vi "Puff_Analysis_AN.vi"(6 "Input Peak":dbl, 7 "Input Own Peak Value?":bool, 8 "Concentration":dbl[](array[numeric]), 9 "Time":dbl[](array[numeric])) -> (0 "End Index":i32, 1 "Start Index":i32, 2 "Channel Values":string[](array[string]), 3 "Channel Names":string[](array[string]))   [LabVIEW 2022 SP3]
uses:
  <vilib>/Analysis/6fits.llb/Curve Fitting Criteria.ctl
  <vilib>/Analysis/baseanly.llb/Mean (DBL).vi
  <vilib>/Analysis/NI_AALBase.lvlib
  <vilib>/Analysis/NI_AALPro.lvlib
panel:
  out "% Error":dbl
  out "offset":dbl
  out "Decay Constant (s)":dbl
  out "Start":dbl
  out "End":dbl
  out "XY Graph":cluster{"Time":dbl[], "Concentration":dbl[]}[](graph)
  out "Decay Time":dbl
  out "50-50 Time":dbl
  out "Rise Time":dbl
  out "Fall Times":dbl[](array[numeric])
  out "Rise Times":dbl[](array[numeric])
  out "Peak Value":dbl
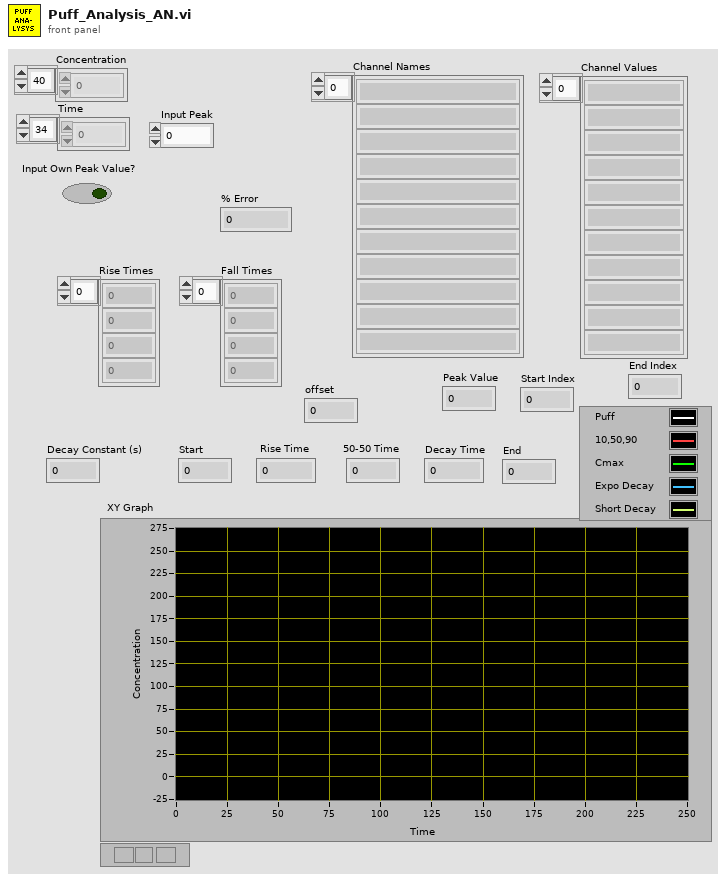
[diagram p1: front panel]
types:
  T1 = cluster{"amp min":dbl, "amp max":dbl, "damping min":dbl, "damping max":dbl, "offset min":dbl, "offset max":dbl}
  T2 = typedef "NI_AALPro.lvlib/Curve Fitting Criteria.ctl" = u16
  T3 = cluster{"Time":dbl[], "Best Exponential Fit":dbl[]}[]
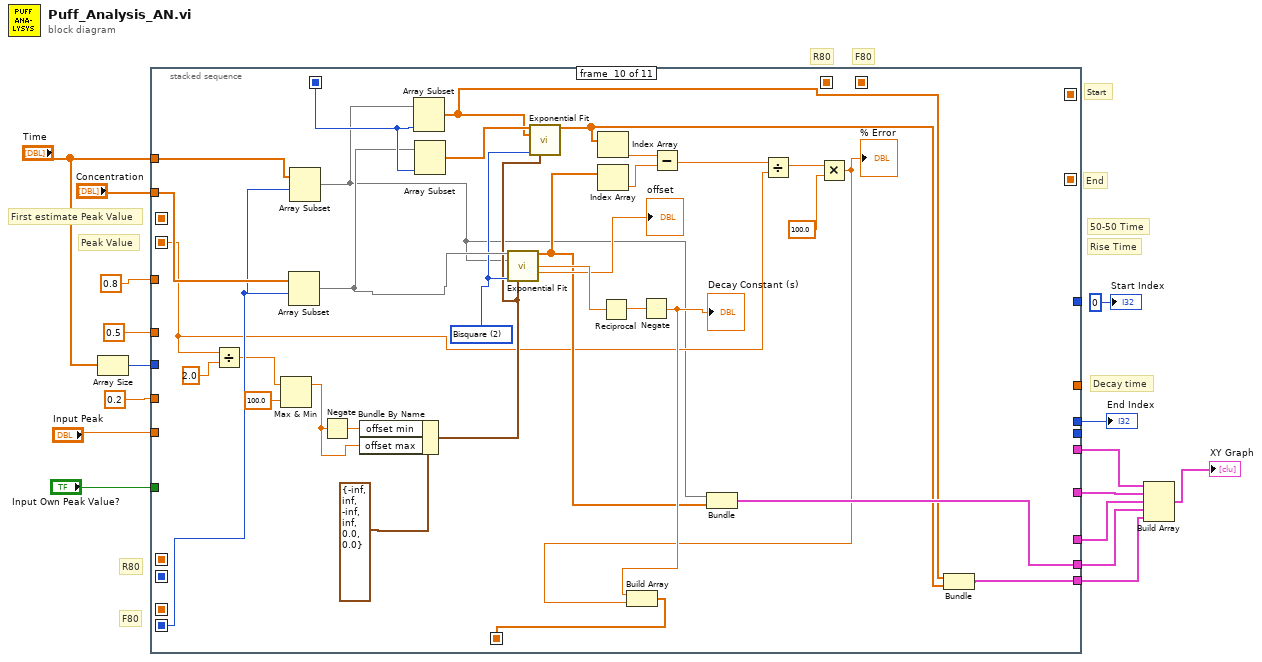
[diagram p0: block diagram]
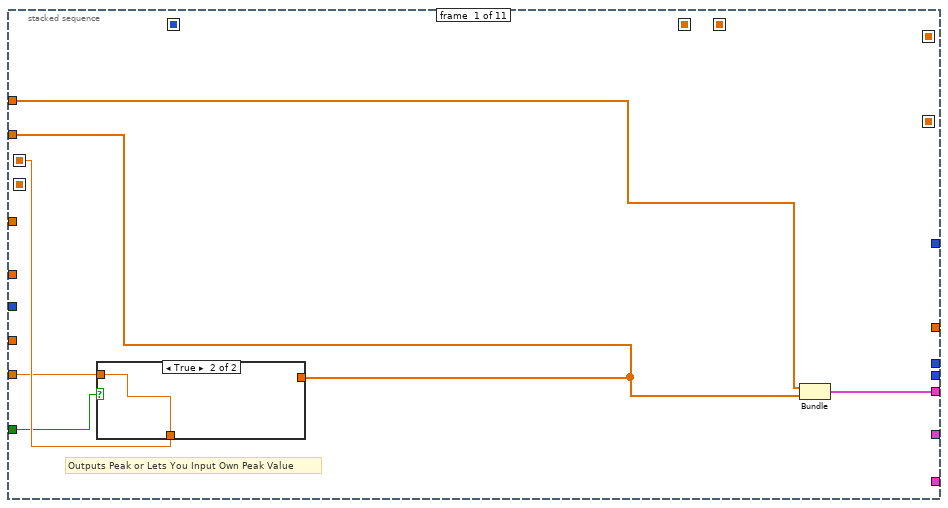
[diagram p2: hidden frame]
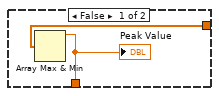
[diagram p3: hidden frame]
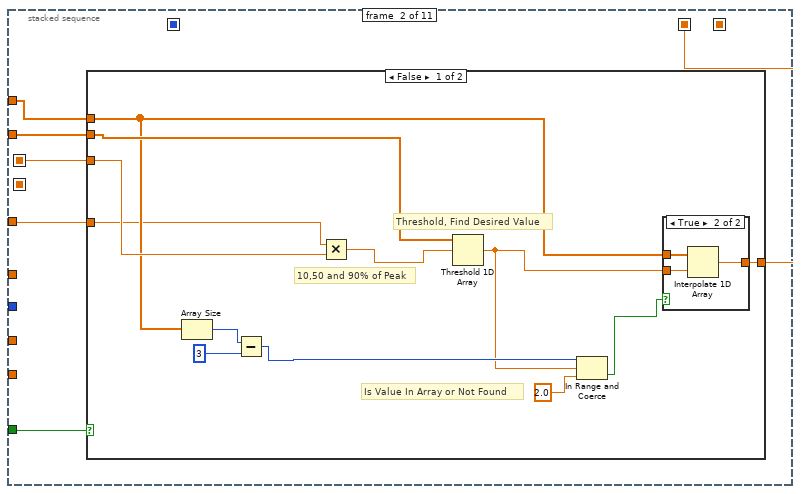
[diagram p4: hidden frame]
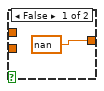
[diagram p5: hidden frame]
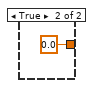
[diagram p6: hidden frame]
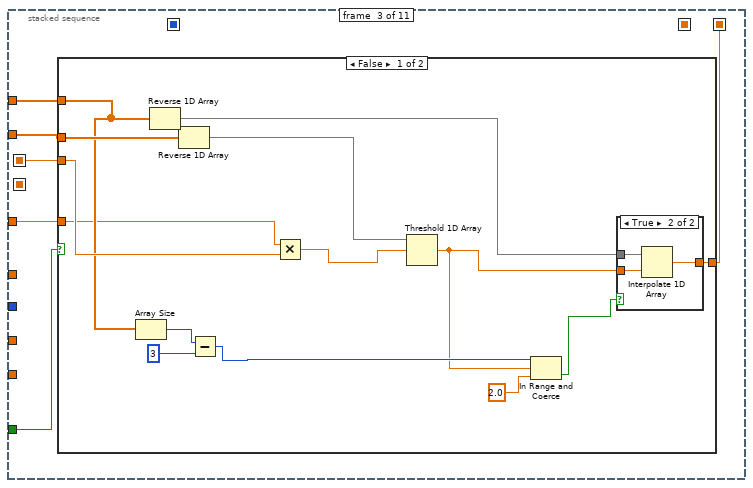
[diagram p7: hidden frame]
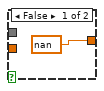
[diagram p8: hidden frame]
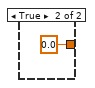
[diagram p9: hidden frame]
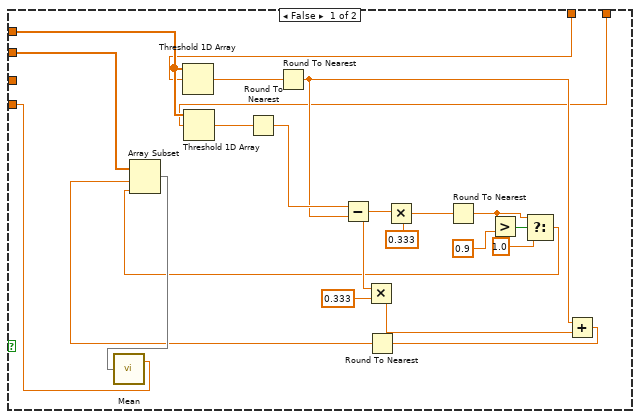
[diagram p11: hidden frame]
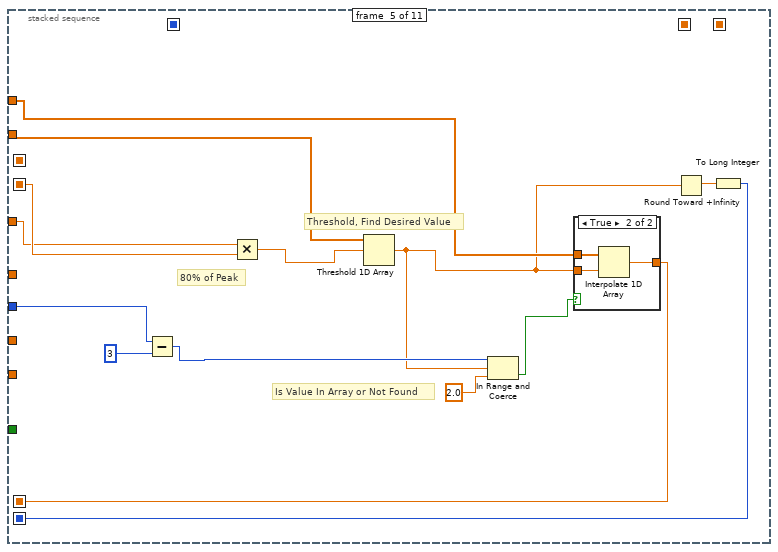
[diagram p12: hidden frame]
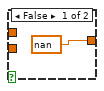
[diagram p13: hidden frame]
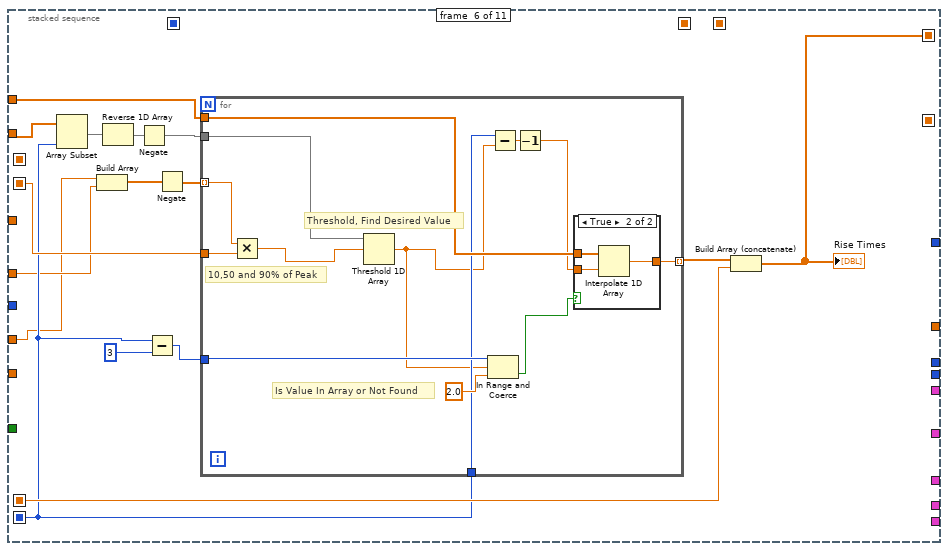
[diagram p14: hidden frame]
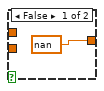
[diagram p15: hidden frame]
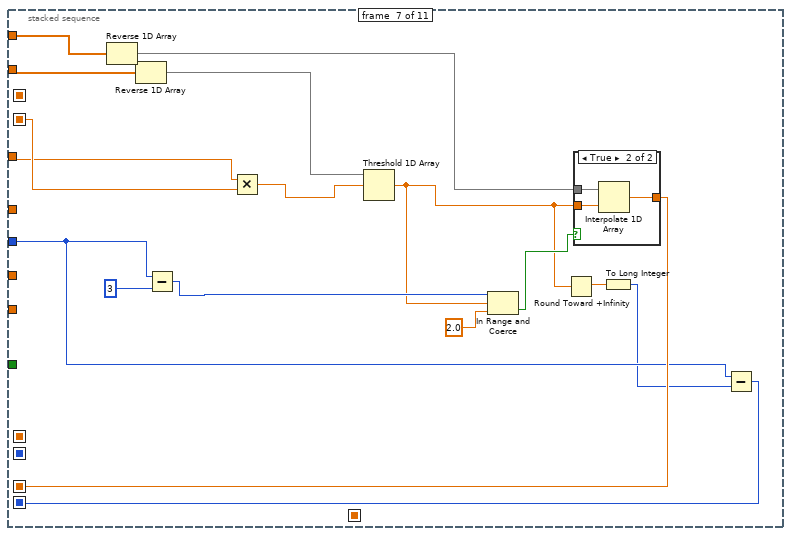
[diagram p16: hidden frame]
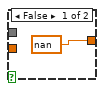
[diagram p17: hidden frame]
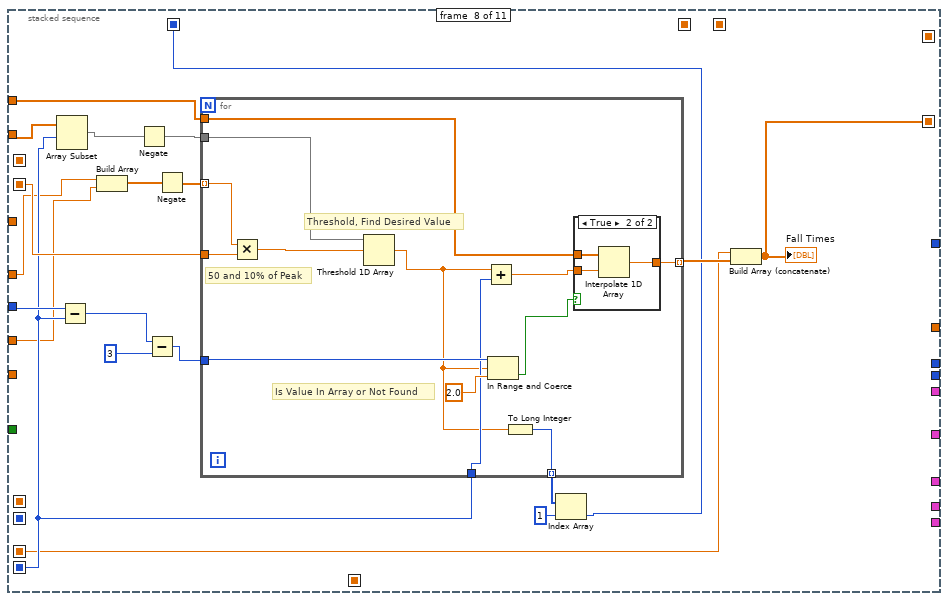
[diagram p18: hidden frame]
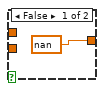
[diagram p19: hidden frame]
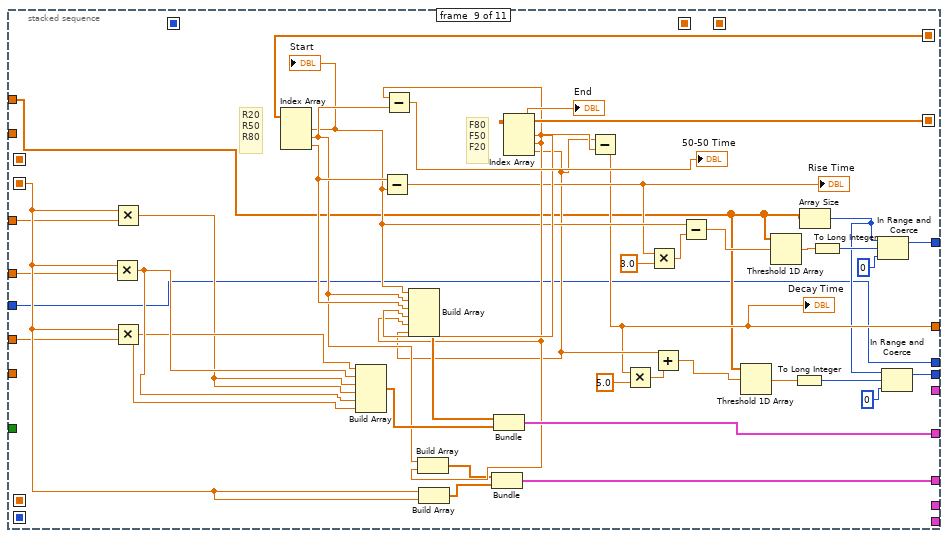
[diagram p20: hidden frame]
diagram:
  # "F80"
  # "R80"
  # "Peak Value"
  # "F80"
  # "R80"
  # "Decay time"
  # "Rise Time"
  # "50-50 Time"
  # "End"
  # "Start"
  # "First estimate Peak Value"
  n1 = Array Size(array="Time") -> (size(s)=w8:i32)
  n2 = stacked-sequence {
    seq-local: [w22 _ _ _ _ _ _ _ _ _ _] -> [_ w31 w54 w78 _ _ _ _ _ _ _]
    seq-local: [_ _ _ _ _ w127 _ _ _ _ _] -> [_ _ _ _ _ _ _ _ w253 _ w311]
    seq-local: [_ _ _ _ _ _ _ w185 _ _ _] -> [_ _ _ _ _ _ _ _ w252 _ w310]
    seq-local: [_ w28 _ _ _ _ _ _ _ _ _] -> [_ _ _ w75 _ _ _ _ _ _ _]
    seq-local: [_ _ w51 _ _ _ _ _ _ _ _] -> [_ _ _ w74 _ _ _ _ _ _ _]
    seq-local: [_ _ _ w79 _ _ _ _ _ _ _] -> [_ _ _ _ w113 w135 w165 w193 w237 w261 w291]
    seq-local: [_ _ _ _ w108 _ _ _ _ _ _] -> [_ _ _ _ _ w126 _ _ _ _ _]
    seq-local: [_ _ _ _ w106 _ _ _ _ _ _] -> [_ _ _ _ _ w124 _ _ _ _ _]
    seq-local: [_ _ _ _ _ _ w161 _ _ _ _] -> [_ _ _ _ _ _ _ w181 _ _ _]
    seq-local: [_ _ _ _ _ _ w156 _ _ _ _] -> [_ _ _ _ _ _ _ w183 _ w280 _]
    seq-local: [_ _ _ _ _ _ _ _ _ w272 _] -> [_ _ _ _ _ _ _ _ _ _ w287]
    seq-local: [_ _ _ _ _ _ _ w177 _ _ _] -> [_ _ _ _ _ _ _ _ _ w270 _]
    tunnel: [_ _ _ _ _ _ _ _ w227 _ _] -> _
    tunnel: [w21 _ _ _ _ _ _ _ _ _ _] -> w16
    tunnel: [_ _ _ _ _ _ _ _ w244 _ _] -> w14
    tunnel: [_ _ _ _ _ _ _ _ w238 _ _] -> w13
    tunnel: "Time" -> [w20 w29 w52 w76 w114 w128 w166 w188 w221 w271 _]
    tunnel: "Concentration" -> [w19 w30 w53 w77 w115 w129 w167 w189 _ w285 _]
    tunnel: "Input Own Peak Value?" -> [w18 w27 w50 w80 _ _ _ _ _ _ w295]
    tunnel: "Input Peak" -> [w17 _ _ _ _ _ _ _ _ _ _]
    tunnel: w8 -> [_ _ _ _ w109 _ w158 w184 w213 _ _]
    tunnel: 0.8 ("y") -> [_ w26 w49 _ w104 _ w155 _ w236 _ _]
    tunnel: 0.2 ("y") -> [_ _ _ _ _ w122 _ w180 w235 _ _]
    tunnel: 0.5 ("y") -> [_ _ _ _ _ w123 _ w179 w234 _ _]
    tunnel: [_ _ _ _ _ _ _ _ w218 _ _] -> _
    tunnel: [_ _ _ _ _ _ _ _ w214 _ _] -> _
    tunnel: [_ _ _ _ _ _ _ _ w213 _ _] -> w3
    tunnel: [_ _ _ _ _ _ _ _ _ w274 _] -> w2
    tunnel: [_ _ _ _ _ _ _ _ _ w254 _] -> w1
    frame #0 {
      # "Outputs Peak or Lets You Input Own Peak Value"
      n3 = case shown="True" w18 {
        tunnel: [w24 w25] -> w22
        tunnel: w19 -> [w23 _]
        tunnel: w17 -> [_ w25]
        frame False {
          n4 = Array Max & Min(array=w23) -> (max value=w24:dbl)  [unwired: 3 out]
          "Peak Value" <- w24
        }
        frame True {
        }
      }
      n5 = Bundle("Time"=w20, "Concentration"=w19) -> (w21:cluster{"Time":dbl[], "Concentration":dbl[]})  [unwired: 1 in]
    }
    frame #1 {
      n6 = case shown="False" w27 {
        tunnel: w31 -> [w43 _]
        tunnel: w30 -> [w39 _]
        tunnel: w29 -> [w38 _]
        tunnel: [w37 0.0] -> w28
        tunnel: w26 -> [w32 _]
        frame False {
          # "10,50 and 90% of Peak"
          # "Is Value In Array or Not Found"
          # "Threshold, Find Desired Value"
          n7 = Array Size(array=w38) -> (size(s)=w41:i32)
          n8 = Subtract(x=w41, y=3) -> (x-y=w40:i32)
          n9 = Multiply(x=w32, y=w43) -> (x*y=w36:dbl)
          n10 = Threshold 1D Array(2:w36, 3:w39) -> (0:w33:dbl)  [unwired: 1 in]
          n11 = In Range and Coerce(upper limit=w40, x=w33, lower limit=2.0) -> (In Range?=w34:bool)  [unwired: 1 out]
          n12 = case shown="True" w34 {
            tunnel: w33 -> [_ w47]
            tunnel: [nan w46] -> w37
            tunnel: w38 -> [_ w45]
            frame False {
            }
            frame True {
              n13 = Interpolate 1D Array(1:w47, 2:w45) -> (0:w46:dbl)
            }
          }
        }
        frame True {
        }
      }
    }
    frame #2 {
      n14 = case shown="False" w50 {
        tunnel: w54 -> [w68 _]
        tunnel: w53 -> [w62 _]
        tunnel: w52 -> [w61 _]
        tunnel: [w57 0.0] -> w51
        tunnel: w49 -> [w56 _]
        frame False {
          n15 = Array Size(array=w61) -> (size(s)=w66:i32)
          n16 = Reverse 1D Array(array=w61) -> (reversed array=w64:dbl[])
          n17 = Reverse 1D Array(array=w62) -> (reversed array=w63:dbl[])
          n18 = Subtract(x=w66, y=3) -> (x-y=w65:i32)
          n19 = Multiply(x=w56, y=w68) -> (x*y=w60:dbl)
          n20 = Threshold 1D Array(2:w60, 3:w63) -> (0:w55:dbl)  [unwired: 1 in]
          n21 = In Range and Coerce(upper limit=w65, x=w55, lower limit=2.0) -> (In Range?=w58:bool)  [unwired: 1 out]
          n22 = case shown="True" w58 {
            tunnel: w55 -> [_ w72]
            tunnel: [nan w71] -> w57
            tunnel: w64 -> [_ w70]
            frame False {
            }
            frame True {
              n23 = Interpolate 1D Array(1:w72, 2:w70) -> (0:w71:dbl)
            }
          }
        }
        frame True {
        }
      }
    }
    frame #3 {
      n24 = case shown="True" w80 {
        tunnel: [w89 w103] -> w79
        tunnel: w78 -> [_ w103]
        tunnel: w77 -> [w102 _]
        tunnel: w76 -> [w100 _]
        tunnel: w75 -> [w88 _]
        tunnel: w74 -> [w87 _]
        frame False {
          n25 = Threshold 1D Array(2:w88, 3:w100) -> (0:w101:dbl)  [unwired: 1 in]
          n26 = Threshold 1D Array(2:w87, 3:w100) -> (0:w99:dbl)  [unwired: 1 in]
          n27 = Round To Nearest(number=w99) -> (nearest integer value=w98:dbl)
          n28 = Round To Nearest(number=w101) -> (nearest integer value=w92:dbl)
          n29 = Subtract(x=w98, y=w92) -> (x-y=w95:dbl)
          n30 = Multiply(x=w95, y=0.333) -> (x*y=w93:dbl)
          n31 = Multiply(x=w95, y=0.333) -> (x*y=w96:dbl)
          n32 = Round To Nearest(number=w96) -> (nearest integer value=w83:dbl)
          n33 = Greater?(x=w83, y=0.9) -> (0:w84:bool)
          n34 = Select(t=w83, s=w84, f=1.0) -> (s? t:f=w81:dbl)
          n35 = Add(x=w92, y=w93) -> (x+y=w91:dbl)
          n36 = Round To Nearest(number=w91) -> (nearest integer value=w86:dbl)
          n37 = Array Subset(array=w102, index=w86, length=w81) -> (w90:dbl[])
          n38 = call-poly <vilib>:"Mean.vi"("X"=w90) -> ("mean"=w89:dbl)  [unwired: 1 out]
        }
        frame True {
        }
      }
    }
    frame #4 {
      # "80% of Peak"
      # "Is Value In Array or Not Found"
      # "Threshold, Find Desired Value"
      n39 = Subtract(x=w109, y=3) -> (x-y=w116:i32)
      n40 = Multiply(x=w104, y=w113) -> (x*y=w112:dbl)
      n41 = Threshold 1D Array(2:w112, 3:w115) -> (0:w105:dbl)  [unwired: 1 in]
      n42 = In Range and Coerce(upper limit=w116, x=w105, lower limit=2.0) -> (In Range?=w110:bool)  [unwired: 1 out]
      n43 = case shown="True" w110 {
        tunnel: w105 -> [_ w121]
        tunnel: [nan w120] -> w108
        tunnel: w114 -> [_ w119]
        frame False {
        }
        frame True {
          n44 = Interpolate 1D Array(1:w121, 2:w119) -> (0:w120:dbl)
        }
      }
      n45 = Round Toward +Infinity(x=w105) -> (ceil(x): smallest int >= x=w107:dbl)
      n46 = To Long Integer(number=w107) -> (32bit integer=w106:i32)
    }
    frame #5 {
      n47 = Array Subset(array=w129, length=w124) -> (w134:dbl[])  [unwired: 1 in]
      n48 = Build Array(w122, w123) -> (w132:dbl[])
      n49 = Reverse 1D Array(array=w134) -> (reversed array=w133:dbl[])
      n50 = Negate(x=w133) -> (-x=w130:dbl[])
      n51 = Subtract(x=w124, y=3) -> (x-y=w136:i32)
      n52 = Negate(x=w132) -> (-x=w131:dbl[])
      n53 = for {
        tunnel: w131 -> [w148] mode=indexing
        tunnel: w135 -> [w149]
        tunnel: w128 -> [w145]
        tunnel: w130 -> [w146]
        tunnel: [w147] -> w125 mode=indexing
        tunnel: w136 -> [w144]
        tunnel: w124 -> [w141]
        # "10,50 and 90% of Peak"
        # "Is Value In Array or Not Found"
        # "Threshold, Find Desired Value"
        n54 = Multiply(x=w148, y=w149) -> (x*y=w150:dbl)
        n55 = Threshold 1D Array(2:w150, 3:w146) -> (0:w140:dbl)  [unwired: 1 in]
        n56 = In Range and Coerce(upper limit=w144, x=w140, lower limit=2.0) -> (In Range?=w142:bool)  [unwired: 1 out]
        n57 = Subtract(x=w141, y=w140) -> (x-y=w139:dbl)
        n58 = Decrement(x=w139) -> (x-1=w138:dbl)
        n59 = case shown="True" w142 {
          tunnel: w138 -> [_ w154]
          tunnel: [nan w153] -> w147
          tunnel: w145 -> [_ w152]
          frame False {
          }
          frame True {
            n60 = Interpolate 1D Array(1:w154, 2:w152) -> (0:w153:dbl)
          }
        }
      }
      n61 = Build Array (concatenate)(w125, w126) -> (w127:dbl[])
      "Rise Times" <- w127
    }
    frame #6 {
      n62 = Reverse 1D Array(array=w166) -> (reversed array=w169:dbl[])
      n63 = Reverse 1D Array(array=w167) -> (reversed array=w168:dbl[])
      n64 = Subtract(x=w158, y=3) -> (x-y=w170:i32)
      n65 = Multiply(x=w155, y=w165) -> (x*y=w164:dbl)
      n66 = Threshold 1D Array(2:w164, 3:w168) -> (0:w159:dbl)  [unwired: 1 in]
      n67 = In Range and Coerce(upper limit=w170, x=w159, lower limit=2.0) -> (In Range?=w162:bool)  [unwired: 1 out]
      n68 = Round Toward +Infinity(x=w159) -> (ceil(x): smallest int >= x=w160:dbl)
      n69 = case shown="True" w162 {
        tunnel: w159 -> [_ w175]
        tunnel: [nan w174] -> w161
        tunnel: w169 -> [_ w173]
        frame False {
        }
        frame True {
          n70 = Interpolate 1D Array(1:w175, 2:w173) -> (0:w174:dbl)
        }
      }
      n71 = To Long Integer(number=w160) -> (32bit integer=w157:i32)
      n72 = Subtract(x=w158, y=w157) -> (x-y=w156:i32)
    }
    frame #7 {
      n73 = Array Subset(array=w189, index=w183) -> (w186:dbl[])  [unwired: 1 in]
      n74 = Subtract(x=w184, y=w183) -> (x-y=w182:i32)
      n75 = Build Array(w179, w180) -> (w192:dbl[])
      n76 = Negate(x=w186) -> (-x=w190:dbl[])
      n77 = Subtract(x=w182, y=3) -> (x-y=w194:i32)
      n78 = Negate(x=w192) -> (-x=w191:dbl[])
      n79 = for {
        tunnel: w191 -> [w206] mode=indexing
        tunnel: w193 -> [w207]
        tunnel: w188 -> [w203]
        tunnel: w190 -> [w204]
        tunnel: [w205] -> w187 mode=indexing
        tunnel: w194 -> [w202]
        tunnel: w183 -> [w199]
        tunnel: [w197] -> w178 mode=indexing
        # "50 and 10% of Peak"
        # "Is Value In Array or Not Found"
        # "Threshold, Find Desired Value"
        n80 = Multiply(x=w206, y=w207) -> (x*y=w208:dbl)
        n81 = Threshold 1D Array(2:w208, 3:w204) -> (0:w196:dbl)  [unwired: 1 in]
        n82 = Add(x=w196, y=w199) -> (x+y=w198:dbl)
        n83 = In Range and Coerce(upper limit=w202, x=w196, lower limit=2.0) -> (In Range?=w200:bool)  [unwired: 1 out]
        n84 = To Long Integer(number=w196) -> (32bit integer=w197:i32)
        n85 = case shown="True" w200 {
          tunnel: w198 -> [_ w212]
          tunnel: [nan w211] -> w205
          tunnel: w203 -> [_ w210]
          frame False {
          }
          frame True {
            n86 = Interpolate 1D Array(1:w212, 2:w210) -> (0:w211:dbl)
          }
        }
      }
      n87 = Index Array(array=w178, index=1) -> (element=w177:i32)
      n88 = Build Array (concatenate)(w181, w187) -> (w185:dbl[])
      "Fall Times" <- w185
    }
    frame #8 {
      # "R20\nR50\nR80"
      # "F80\nF50\nF20"
      n89 = Multiply(x=w237, y=w234) -> (x*y=w250:dbl)
      n90 = Multiply(x=w237, y=w236) -> (x*y=w241:dbl)
      n91 = Multiply(x=w237, y=w235) -> (x*y=w249:dbl)
      n92 = Index Array(array=w253) -> (element #1=w233:dbl, element #2=w243:dbl, element #3=w248:dbl)  [unwired: 3 in]
      "Start" <- w233
      n93 = Build Array(w249, w250, w241, w241, w250, w249) -> (w245:dbl[])
      n94 = Subtract(x=w248, y=w233) -> (x-y=w230:dbl)
      "Rise Time" <- w230
      n95 = Build Array(w237, w237) -> (w240:dbl[])
      n96 = Index Array(array=w252) -> (element #1=w247:dbl, element #2=w242:dbl, element #3=w229:dbl)  [unwired: 3 in]
      "End" <- w247
      n97 = Subtract(x=w242, y=w243) -> (x-y=→"50-50 Time":dbl)
      n98 = Build Array(w233, w243, w248, w247, w242, w229) -> (w246:dbl[])
      n99 = Build Array(w243, w242) -> (w239:dbl[])
      n100 = Bundle(w239, w240) -> (w238:cluster{dbl[], dbl[]})  [unwired: 1 in]
      n101 = Bundle(w246, w245) -> (w244:cluster{dbl[], dbl[]})  [unwired: 1 in]
      n102 = Subtract(x=w229, y=w247) -> (x-y=w227:dbl)
      "Decay Time" <- w227
      n103 = Multiply(x=w227, y=5.0) -> (x*y=w228:dbl)
      n104 = Multiply(x=w230, y=3.0) -> (x*y=w232:dbl)
      n105 = Add(x=w229, y=w228) -> (x+y=w223:dbl)
      n106 = Subtract(x=w233, y=w232) -> (x-y=w225:dbl)
      n107 = Threshold 1D Array(2:w223, 3:w221) -> (0:w222:dbl)  [unwired: 1 in]
      n108 = Threshold 1D Array(2:w225, 3:w221) -> (0:w224:dbl)  [unwired: 1 in]
      n109 = To Long Integer(number=w222) -> (32bit integer=w216:i32)
      n110 = Array Size(array=w221) -> (size(s)=w215:i32)
      n111 = To Long Integer(number=w224) -> (32bit integer=w220:i32)
      n112 = In Range and Coerce(upper limit=w215, x=w220, lower limit=0) -> (coerced(x)=w218:i32)  [unwired: 1 out]
      n113 = In Range and Coerce(upper limit=w215, x=w216, lower limit=0) -> (coerced(x)=w214:i32)  [unwired: 1 out]
    }
    frame #9 {
      w267 = T2 2 items=["Least Square", "Least Absolute Residual", "Bisquare"] ("method")
      n114 = Divide(x=w261, y=2.0) -> (x/y=w278:dbl)
      n115 = Max & Min(x=w278, y=100.0) -> (max(x,y)=w275:dbl)  [unwired: 1 out]
      n116 = Array Subset(array=w285, index=w280) -> (w269:dbl[])  [unwired: 1 in]
      n117 = Array Subset(array=w271, index=w280) -> (w257:dbl[])  [unwired: 1 in]
      n118 = Negate(x=w275) -> (-x=w276:dbl)
      n119 = Bundle By Name(cluster=T1 {"amp min"=-inf, "amp max"=inf, "damping min"=-inf, "damping max"=inf, "offset min"=0.0, "offset max"=0.0} ("parameter bounds"), "offset min"=w276, "offset max"=w275) -> (w266:T1)
      n120 = Array Subset(array=w257, length=w270) -> (w256:dbl[])  [unwired: 1 in]
      n121 = Array Subset(array=w269, length=w270) -> (w268:dbl[])  [unwired: 1 in]
      n122 = call <vilib>:"Exponential Fit.vi"("Y"=w269, "X"=w257, "method"=w267, "parameter bounds"=w266) -> ("Best Exponential Fit"=w265:dbl[], "damping"=w284:dbl, "offset"=→"offset":dbl)  [unwired: 6 in, 3 out]
      n123 = call <vilib>:"Exponential Fit.vi"("Y"=w268, "X"=w256, "method"=w267, "parameter bounds"=w266) -> ("Best Exponential Fit"=w255:dbl[])  [unwired: 6 in, 5 out]
      n124 = Index Array(array=w255) -> (element=w263:dbl)  [unwired: 1 in]
      n125 = Index Array(array=w265) -> (element=w264:dbl)  [unwired: 1 in]
      n126 = Reciprocal(x=w284) -> (1/x=w283:dbl)
      n127 = Negate(x=w283) -> (-x=w273:dbl)
      "Decay Constant (s)" <- w273
      n128 = Subtract(x=w263, y=w264) -> (x-y=w262:dbl)
      n129 = Bundle(w257, "Best Exponential Fit"=w265) -> (w274:cluster{dbl[], "Best Exponential Fit":dbl[]})  [unwired: 1 in]
      n130 = Divide(x=w262, y=w261) -> (x/y=w260:dbl)
      n131 = Multiply(x=w260, y=100.0) -> (x*y=w258:dbl)
      "% Error" <- w258
      n132 = Build Array(w273, w258) -> (w272:dbl[])
      n133 = Bundle(w256, "Best Exponential Fit"=w255) -> (w254:cluster{dbl[], "Best Exponential Fit":dbl[]})  [unwired: 1 in]
    }
    frame #10 {
      n134 = case shown="False" w295 {
        tunnel: [" Meas Peak" " Supplied Peak"] -> w294
        frame False {
        }
        frame True {
        }
      }
      n135 = Build Array("Value (ppm):of", "Rise Time (s):to 20% of", "Rise Time (s):to 50% of", "Rise Time (s):to 80% of", "Rise Time (s):R80-R20 of", "Time (s):F50-R50 of", "Decay Time (s):F20-F80 of", "Fall Time (s):to 80% of", "Fall Time (s):to 50% of", "Fall Time (s):to 20% of") -> (w293:string[])
      n136 = for {
        tunnel: w294 -> [w316]
        tunnel: w293 -> [w315] mode=indexing
        tunnel: [w314] -> w290 mode=indexing
        n137 = Concatenate Strings(w315, w316) -> (w314:string)
      }
      n138 = local read "Decay Time"() -> (w307:dbl)
      n139 = local read "50-50 Time"() -> (w308:dbl)
      n140 = local read "Rise Time"() -> (w309:dbl)
      n141 = Build Array (concatenate)(w291, w311, w309, w308, w307, w310, w287) -> (w297:dbl[])
      n142 = Number To Fractional String(number=w297) -> (F-format string=→"Channel Values":string[])  [unwired: 3 in]
      n143 = Build Array (concatenate)(w290, "Expo Decay:Time (s)", "Expo Decay:% Fit Error") -> (→"Channel Names":string[])
    }
  }
  "End Index" <- w3
  n144 = Build Array(w16, w14, w13, w2, w1) -> (→"XY Graph":T3)
  "Start Index" <- 0 ("Start Index")
